vi "Get Protocol.vi"(8 "error in (no error)":errorcluster, 11 "SessionOptions in":refnum<class "SessionOptions.lvclass">) -> (0 "error out":errorcluster, 2 "Protocol":T1=1 items=["Sftp", "Scp", "Ftp", "Webdav", "S3"], 3 "SessionOptions out":refnum<class "SessionOptions.lvclass">)   [LabVIEW 2015, in "SessionOptions.lvclass"]
uses:
  SessionOptions.lvclass
  Protocols--Ring.ctl
  SessionOptions.lvclass/SessionOptions.ctl
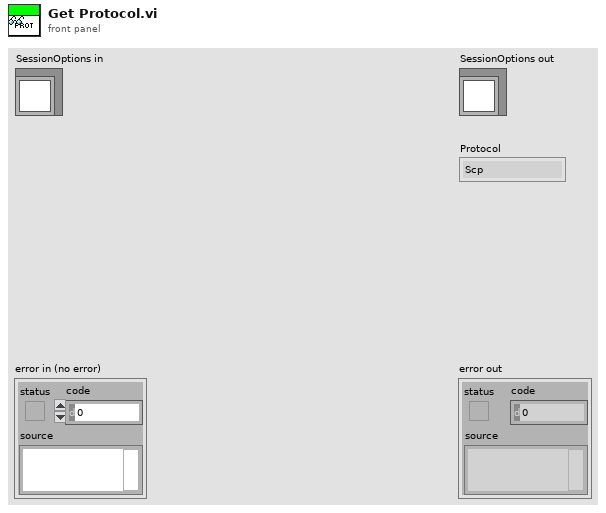
[diagram p1: front panel]
types:
  T1 = typedef "SessionOptions.lvclass/Protocols--Ring.ctl" = i32
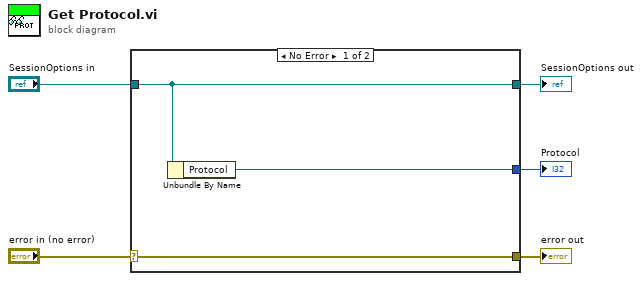
[diagram p0: block diagram]
diagram:
  n1 = case shown="No Error" "error in (no error)" {
    selector: "error in (no error)" -> [w8 w9]
    tunnel: [w8 w9] -> w4
    tunnel: [w7 w10] -> w2
    tunnel: "SessionOptions in" -> [w7 w10]
    tunnel: [w6 _] -> w1
    frame No Error {
      n2 = Unbundle By Name(w7) -> ("Protocol"=w6:T1)
    }
    frame Error {
    }
  }
  "error out" <- w4
  "SessionOptions out" <- w2
  "Protocol" <- w1
